vi "Mqtt_Decode_CMD1_Content.vi"(8 "error in (no error)":errorcluster, 11 "jsContent":string) -> (0 "error out":errorcluster, 3 "clusterContent":T1)   [LabVIEW 2020]
uses:
  <vilib>/addons/JSON API/JSON Value/Set from JSON string.vi
  <vilib>/addons/JSON API/JSON Value/Get Object Item by Name.vi
  <vilib>/addons/JSON API/JSON Scalar/Get as Text.vi
  <vilib>/addons/JSON API/JSON Value/JSON Value.lvclass
  <vilib>/addons/JSON API/Get Polymorphic/JSON GetSet.lvlib
  <vilib>/addons/JSON API/JSON Scalar/JSON Scalar.lvclass
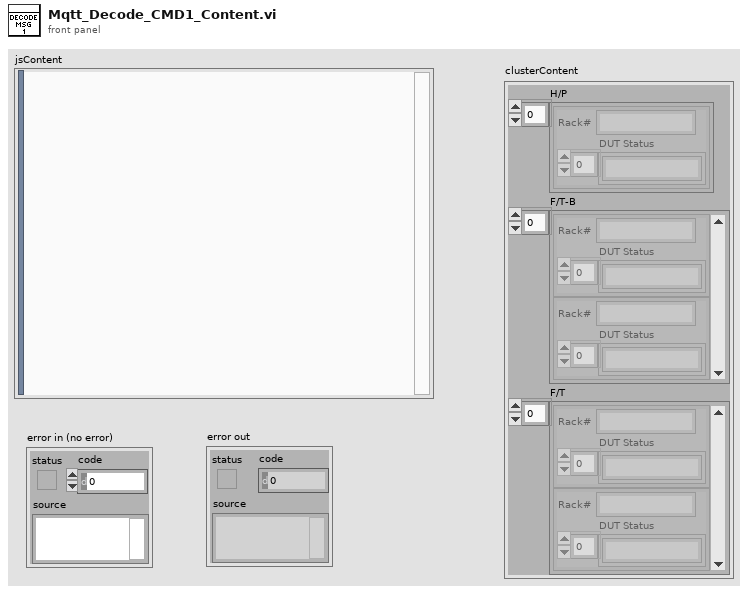
[diagram p1: front panel]
types:
  T1 = cluster{"H/P":cluster{"Rack#":string, "DUT Status":string[]}[], "F/T-B":cluster{"Rack#":string, "DUT Status":string[]}[], "F/T":cluster{"Rack#":string, "DUT Status":string[]}[]}
  T2 = cluster{cluster{string, string[]}[], cluster{string, string[]}[], cluster{string, string[]}[]}
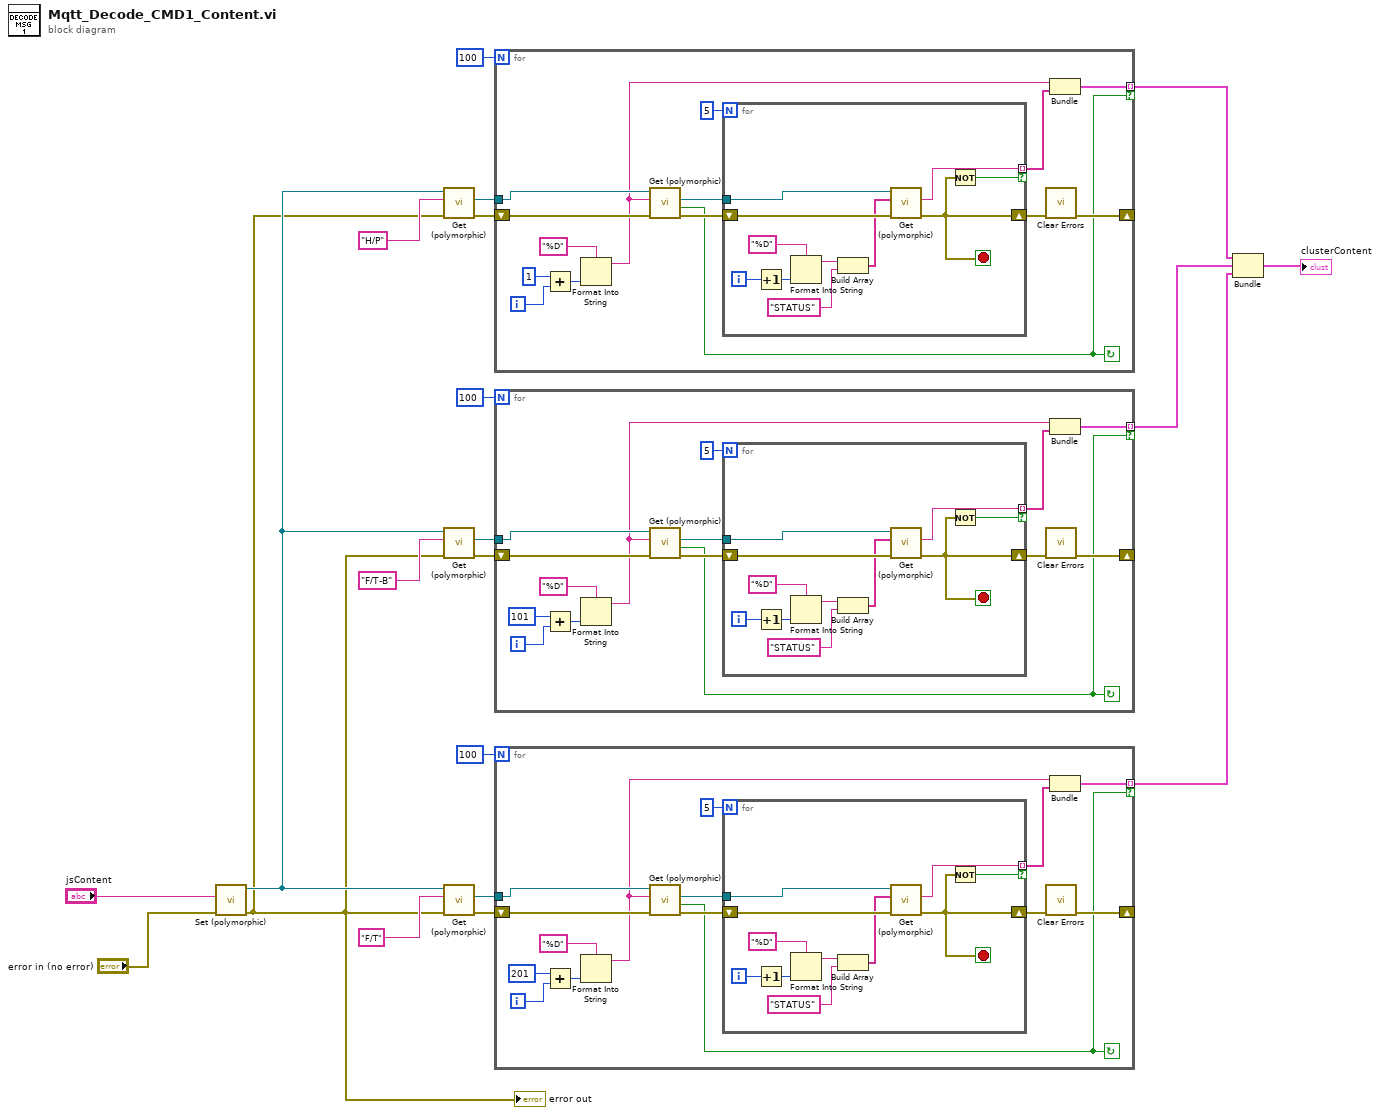
[diagram p0: block diagram]
diagram:
  n1 = call-poly <vilib>:"Set (polymorphic).vi"("error in (no error)"="error in (no error)", "JSON stream"="jsContent") -> ("error out"=w1:errorcluster, "JSON Value out"=w7:refnum<class "JSON Value.lvclass">)  [unwired: 7 in, 1 out]
  "error out" <- w1
  n2 = call-poly <vilib>:"Get (polymorphic).vi"("error in (no error)"=w1, "name"="H/P", "JSON Value In"=w7) -> ("error out"=w8:errorcluster, "Value"=w11:refnum<class "JSON Value.lvclass">)  [unwired: 5 in, 2 out]
  n3 = call-poly <vilib>:"Get (polymorphic).vi"("error in (no error)"=w1, "name"="F/T-B", "JSON Value In"=w7) -> ("error out"=w15:errorcluster, "Value"=w12:refnum<class "JSON Value.lvclass">)  [unwired: 5 in, 2 out]
  n4 = call-poly <vilib>:"Get (polymorphic).vi"("error in (no error)"=w1, "name"="F/T", "JSON Value In"=w7) -> ("error out"=w16:errorcluster, "Value"=w19:refnum<class "JSON Value.lvclass">)  [unwired: 5 in, 2 out]
  n5 = for {
    N: 100 -> [_]
    tunnel: w11 -> [w32]
    shift-right: [w26] -> _
    shift-left: w8 -> [w31]
    tunnel: [w23] -> w6 mode=indexing if=w22
    i -> [w35]
    stop <- w22 continue-if-true
    n6 = Add(x=1, y=w35) -> (x+y=w34:i32)
    n7 = Format Into String(format string="%D", w34) -> (resulting string=w24:string)  [unwired: 2 in, 1 out]
    n8 = call-poly <vilib>:"Get (polymorphic).vi"("error in (no error)"=w31, "name"=w24, "JSON Value In"=w32) -> ("error out"=w28:errorcluster, "found"=w22:bool, "Value"=w29:refnum<class "JSON Value.lvclass">)  [unwired: 5 in, 1 out]
    n9 = for {
      N: 5 -> [_]
      tunnel: w29 -> [w43]
      shift-right: [w38] -> w27
      shift-left: w28 -> [w42]
      tunnel: [w39] -> w25 mode=indexing if=w37
      i -> [w44]
      stop <- w38 stop-if-true
      n10 = Increment(x=w44) -> (x+1=w46:i32)
      n11 = Format Into String(format string="%D", w46) -> (resulting string=w41:string)  [unwired: 2 in, 1 out]
      n12 = Build Array(w41, "STATUS" ("format string")) -> (w40:string[])
      n13 = call-poly <vilib>:"Get (polymorphic).vi"("error in (no error)"=w42, "Name Array"=w40, "JSON Scalar in"=w43) -> ("error out"=w38:errorcluster, "LabVIEW Text"=w39:string)  [unwired: 6 in, 1 out]
      n14 = Not(x=w38) -> (.not. x?=w37:bool)
    }
    n15 = call <vilib>:"Clear Errors.vi"("error in (no error)"=w27) -> ("error out"=w26:errorcluster)  [unwired: 5 in, 1 out]
    n16 = Bundle(w24, w25) -> (w23:cluster{string, string[]})  [unwired: 1 in]
  }
  n17 = for {
    N: 100 -> [_]
    tunnel: w12 -> [w58]
    shift-right: [w52] -> _
    shift-left: w15 -> [w57]
    tunnel: [w49] -> w5 mode=indexing if=w48
    i -> [w61]
    stop <- w48 continue-if-true
    n18 = Add(x=101, y=w61) -> (x+y=w60:i32)
    n19 = Format Into String(format string="%D", w60) -> (resulting string=w50:string)  [unwired: 2 in, 1 out]
    n20 = call-poly <vilib>:"Get (polymorphic).vi"("error in (no error)"=w57, "name"=w50, "JSON Value In"=w58) -> ("error out"=w54:errorcluster, "found"=w48:bool, "Value"=w55:refnum<class "JSON Value.lvclass">)  [unwired: 5 in, 1 out]
    n21 = for {
      N: 5 -> [_]
      tunnel: w55 -> [w69]
      shift-right: [w64] -> w53
      shift-left: w54 -> [w68]
      tunnel: [w65] -> w51 mode=indexing if=w63
      i -> [w70]
      stop <- w64 stop-if-true
      n22 = Increment(x=w70) -> (x+1=w72:i32)
      n23 = Format Into String(format string="%D", w72) -> (resulting string=w67:string)  [unwired: 2 in, 1 out]
      n24 = Build Array(w67, "STATUS" ("format string")) -> (w66:string[])
      n25 = call-poly <vilib>:"Get (polymorphic).vi"("error in (no error)"=w68, "Name Array"=w66, "JSON Scalar in"=w69) -> ("error out"=w64:errorcluster, "LabVIEW Text"=w65:string)  [unwired: 6 in, 1 out]
      n26 = Not(x=w64) -> (.not. x?=w63:bool)
    }
    n27 = call <vilib>:"Clear Errors.vi"("error in (no error)"=w53) -> ("error out"=w52:errorcluster)  [unwired: 5 in, 1 out]
    n28 = Bundle(w50, w51) -> (w49:cluster{string, string[]})  [unwired: 1 in]
  }
  n29 = for {
    N: 100 -> [_]
    tunnel: w19 -> [w84]
    shift-right: [w78] -> _
    shift-left: w16 -> [w83]
    tunnel: [w75] -> w4 mode=indexing if=w74
    i -> [w87]
    stop <- w74 continue-if-true
    n30 = Add(x=201, y=w87) -> (x+y=w86:i32)
    n31 = Format Into String(format string="%D", w86) -> (resulting string=w76:string)  [unwired: 2 in, 1 out]
    n32 = call-poly <vilib>:"Get (polymorphic).vi"("error in (no error)"=w83, "name"=w76, "JSON Value In"=w84) -> ("error out"=w80:errorcluster, "found"=w74:bool, "Value"=w81:refnum<class "JSON Value.lvclass">)  [unwired: 5 in, 1 out]
    n33 = for {
      N: 5 -> [_]
      tunnel: w81 -> [w95]
      shift-right: [w90] -> w79
      shift-left: w80 -> [w94]
      tunnel: [w91] -> w77 mode=indexing if=w89
      i -> [w96]
      stop <- w90 stop-if-true
      n34 = Increment(x=w96) -> (x+1=w98:i32)
      n35 = Format Into String(format string="%D", w98) -> (resulting string=w93:string)  [unwired: 2 in, 1 out]
      n36 = Build Array(w93, "STATUS" ("format string")) -> (w92:string[])
      n37 = call-poly <vilib>:"Get (polymorphic).vi"("error in (no error)"=w94, "Name Array"=w92, "JSON Scalar in"=w95) -> ("error out"=w90:errorcluster, "LabVIEW Text"=w91:string)  [unwired: 6 in, 1 out]
      n38 = Not(x=w90) -> (.not. x?=w89:bool)
    }
    n39 = call <vilib>:"Clear Errors.vi"("error in (no error)"=w79) -> ("error out"=w78:errorcluster)  [unwired: 5 in, 1 out]
    n40 = Bundle(w76, w77) -> (w75:cluster{string, string[]})  [unwired: 1 in]
  }
  n41 = Bundle(w6, w5, w4) -> (→"clusterContent":T2)  [unwired: 1 in]
